vi "HSV to color.vi"(2 "V (intensity)":dbl format="%.2f", 3 "S (Saturation)":dbl format="%.2f", 4 "H (Hue)":dbl format="%.2f") -> (0 "Color":u32)   [LabVIEW 2022 SP3]
doc: "Author: James Nissen, nissen6@llnl.gov\n\nThis vi converts from HSV (Hue Saturation Value) to an RGB color."
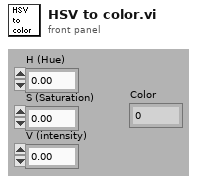
[diagram p1: front panel]
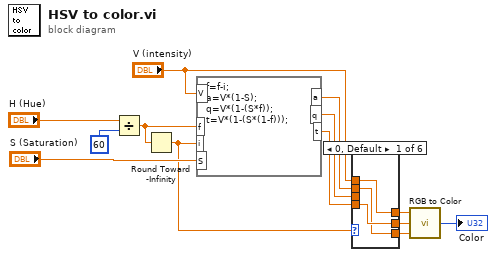
[diagram p0: block diagram]
diagram:
  n1 = Divide(x="H (Hue)", y=60) -> (x/y=w1:dbl)
  n2 = Round Toward -Infinity(1:w1) -> (0:w12:dbl)
  n3 = formula code="f=f-i;\na=V*(1-S);\nq=V*(1-(S*f));\nt=V*(1-(S*(1-f)));"("i"=w12, "S"="S (Saturation)", "V"="V (intensity)", "f"=w1) -> ("a"=w8:dbl, "q"=w9:dbl, "t"=w10:dbl)
  n4 = case shown="0, Default" w12 {
    tunnel: [w16 w19 w22 w25 w28 w31] -> w4
    tunnel: "V (intensity)" -> [w16 w18 w21 w23 w26 w31]
    tunnel: [w15 w18 w21 w24 w27 w30] -> w5
    tunnel: w10 -> [w15 _ w20 _ w28 _]
    tunnel: [w14 w17 w20 w23 w26 w29] -> w6
    tunnel: w8 -> [w14 w17 w22 w25 w27 w30]
    tunnel: w9 -> [_ w19 _ w24 _ w29]
    frame 0, Default {
    }
    frame 1 {
    }
    frame 2 {
    }
    frame 3 {
    }
    frame 4 {
    }
    frame 5 {
    }
  }
  n5 = call <vilib>:"RGB to Color.vi"("B"=w6, "G"=w5, "R"=w4) -> ("Color"=→"Color":u32)
